vi "CmdSetOman_Center2Roi.vi"(8 "yl":i16, 9 "xl":i16, 10 "yc":i16, 11 "xc":i16) -> (2 "roi":string)   [LabVIEW 2016]
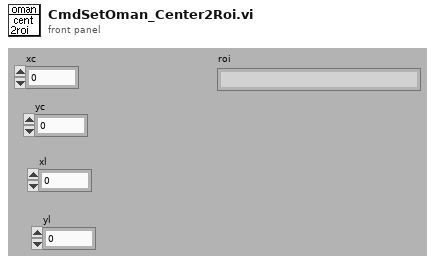
[diagram p1: front panel]
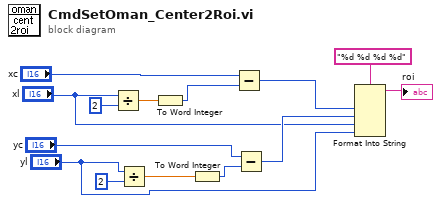
[diagram p0: block diagram]
diagram:
  n1 = Divide(x="xl", y=i16 2) -> (x/y=w12:dbl)
  n2 = Divide(x="yl", y=i16 2) -> (x/y=w9:dbl)
  n3 = To Word Integer(number=w12) -> (16bit integer=w7:i16)
  n4 = To Word Integer(number=w9) -> (16bit integer=w6:i16)
  n5 = Subtract(x="xc", y=w7) -> (x-y=w8:i16)
  n6 = Subtract(x="yc", y=w6) -> (x-y=w5:i16)
  n7 = Format Into String(format string="%d %d %d %d", w8, w5, "xl", "yl") -> (resulting string=→"roi":string)  [unwired: 2 in, 1 out]
